vi "Menu.Properties.Execute.vi"(8 "error in (no error)":errorcluster, 9 "Coords":T3, 10 "ItemTag":string, 11 "Cluster in":T1) -> (0 "error out":errorcluster, 3 "Cluster out":T1)   [LabVIEW 2013, in "Simple Sequence Editor.lvlib"]
uses:
  Simple Sequence Editor.lvlib
  Types/StateVariables.ctl
  Types/ChannelProperties.ctl
  <vilib>/Utility/miscctls.llb/LVPoint32TypeDef.ctl
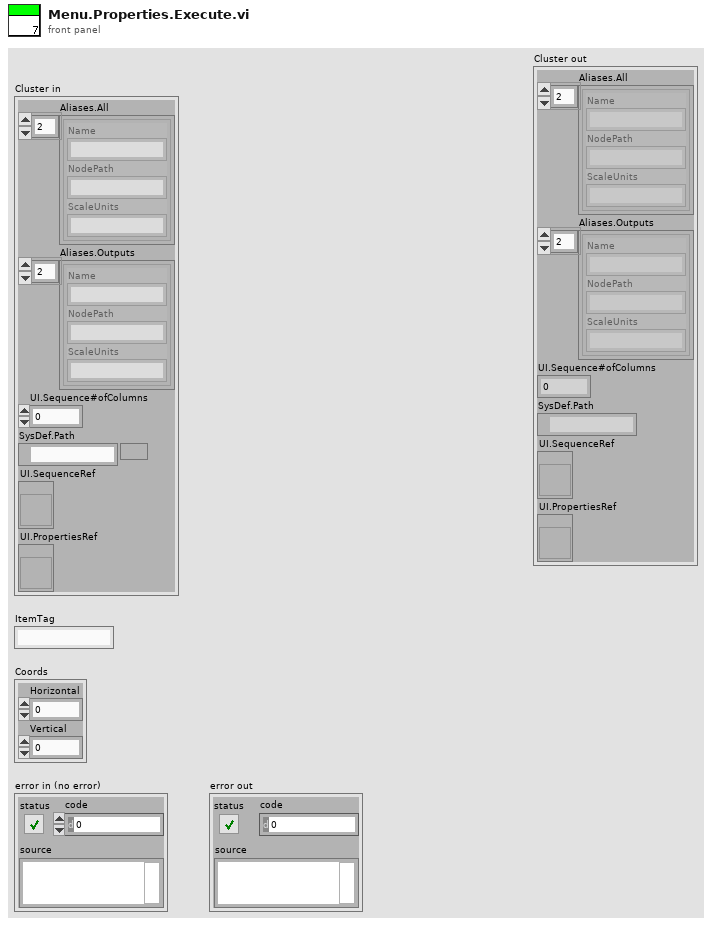
[diagram p1: front panel]
types:
  T1 = typedef "Simple Sequence Editor.lvlib/StateVariables.ctl" = cluster{"Aliases.All":T2[], "Aliases.Outputs":T2[], "UI.Sequence#ofColumns":i32, "SysDef.Path":path, "UI.SequenceRef":refnum<vi>, "UI.PropertiesRef":refnum<vi>}
  T2 = typedef "Simple Sequence Editor.lvlib/ChannelProperties.ctl" = cluster{"Name":string, "NodePath":string, "ScaleUnits":string}
  T3 = typedef "LVPoint32TypeDef.ctl" = cluster{"Horizontal":i32, "Vertical":i32}
  T4 = typedef "LVRowAndColumnTypeDef.ctl" = cluster{"Row":i32, "Column":i32}
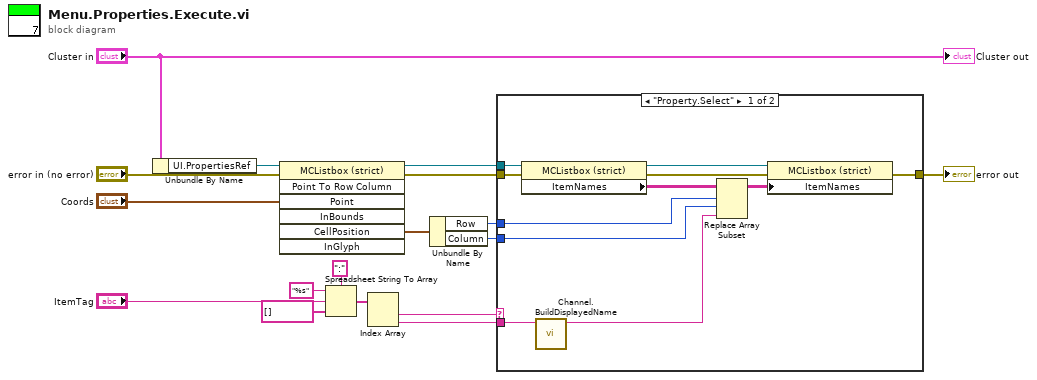
[diagram p0: block diagram]
diagram:
  n1 = Unbundle By Name("Cluster in") -> ("UI.PropertiesRef"=w15:refnum<vi>)
  n2 = invoke class="MCListbox (strict)" method="Point To Row Column"(reference=w15, error in="error in (no error)", "Point"="Coords") -> (reference out=w10:refnum<vi>, error out=w16:errorcluster, "CellPosition"=w11:T4)  [unwired: 4 in, 4 out]
  n3 = Spreadsheet String To Array(delimiter (Tab)=":", format string="%s", spreadsheet string="ItemTag", array type (2D Dbl)=string[] []) -> (array=w3:string[])
  n4 = Index Array(array=w3) -> (element #1=w8:string, element #2=w9:string)  [unwired: 2 in]
  n5 = Unbundle By Name(w11) -> ("Row"=w12:i32, "Column"=w13:i32)
  n6 = case shown="\"Property.Select\"" w8 {
    tunnel: w9 -> [w28 _]
    tunnel: w10 -> [w27 _]
    tunnel: w12 -> [w24 _]
    tunnel: w13 -> [w23 _]
    tunnel: w16 -> [w20 w29]
    tunnel: [w18 w29] -> w17
    frame "Property.Select" {
      n7 = property class="MCListbox (strict)"(reference=w27, error in=w20) -> (reference out=w21:refnum<vi>, error out=w19:errorcluster, "ItemNames"=w26:string[][])
      n8 = call "Channel.BuildDisplayedName.vi"("String in"=w28) -> ("String out"=w25:string)  [unwired: 10 in]
      n9 = Replace Array Subset(array=w26, new element=w25, index (row)=w24, index (col)=w23) -> (w22:string[][])
      n10 = property class="MCListbox (strict)"(reference=w21, error in=w19, "ItemNames"=w22) -> (error out=w18:errorcluster)  [unwired: 1 out]
    }
    frame Default {
    }
  }
  "error out" <- w17
  "Cluster out" <- "Cluster in"
